vi "Error_log.vi"(6 "Clear error?":bool, 8 "error in":errorcluster) -> (0 "error out":errorcluster)   [LabVIEW 2017]
doc: "This SubVI create new or add to existing text file (error_log.txt) data about occured error and current timestamp. Also user can clear occured error by boolean control \"Clear?\"."
uses:
  <vilib>/ErrorRing/Error Ring.xnode
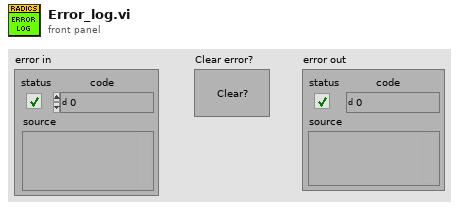
[diagram p1: front panel]
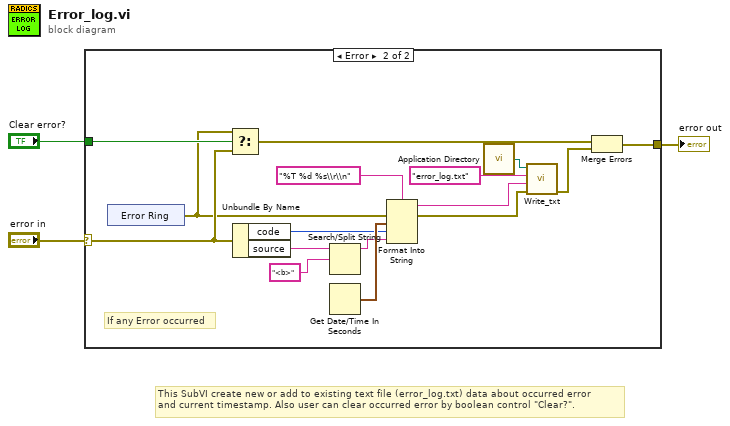
[diagram p0: block diagram]
diagram:
  # "This SubVI create new or add to existing text file (error_log.txt) data about occurred error \nand current timestamp. Also user can clear occurred error by boolean control \"Clear?\"."
  n1 = case shown="Error" "error in" {
    selector: "error in" -> [w4 w12]
    tunnel: [w4 w13] -> w3
    tunnel: "Clear error?" -> [_ w11]
    frame No Error {
      # "If NO Error occurred"
    }
    frame Error {
      # "If any Error occurred"
      n2 = xnode "Error Ring"() -> ("error out"=w5:errorcluster)
      n3 = Select(t=w5, s=w11, f=w12) -> (s? t:f=w14:errorcluster)
      n4 = Unbundle By Name(w12) -> ("code"=w18:i32, "source"=w17:string)
      n5 = Search/Split String(string=w17, search string/char (-)="<b>" ("regular expression")) -> (substring before match=w15:string)  [unwired: 1 in, 2 out]
      n6 = Get Date/Time In Seconds() -> (seconds since 1Jan1904=w19:timestamp)
      n7 = Format Into String(format string="%T %d %s\\r\\n", error in=w5, w19, w18, w15) -> (resulting string=w7:string, error out=w9:errorcluster)  [unwired: 1 in]
      n8 = call <vilib>:"Application Directory.vi"() -> ("Application Directory"=w10:path)
      n9 = call "Write_txt.vi"("error in"=w9, "text"=w7, "filename.txt"="error_log.txt" ("name or relative path"), "base path"=w10) -> ("error out"=w6:errorcluster)  [unwired: 7 in]
      n10 = Merge Errors(w14, w6) -> (w13:errorcluster)
    }
  }
  "error out" <- w3
